vi "calc max motor speed.vi"(10 "DRIVE\nwheel diam (in)":dbl, 11 "swerve motor":T1 {"gear ratio" format="%_5f"; "MOTOR SELECT" items=["REV NEO"=5676, "REV NEO 550"=11000, "VEX Falcon"=6380, "WC Kraken"=6000]}) -> (2 "mav vel (fps)":dbl, 3 "max rpm":dbl)   [LabVIEW 2023]
uses:
  ctrl defs/ctrl swerve motor.ctl
  ctrl defs/ctrl MOTOR SELECT.ctl
  <vilib>/Rock Robotics/WPI/ThirdParty/REV Robotics/REVLib/Typedef/Spark MAX Idle Mode.ctl
  ctrl defs/ctrl Spark MAX current limiting.ctl
  ctrl defs/ctrl motor PIDF coefficients.ctl
  <vilib>/Rock Robotics/WPI/ThirdParty/REV Robotics/REVLib/Typedef/Spark MAX Smart Motion Parameters.ctl
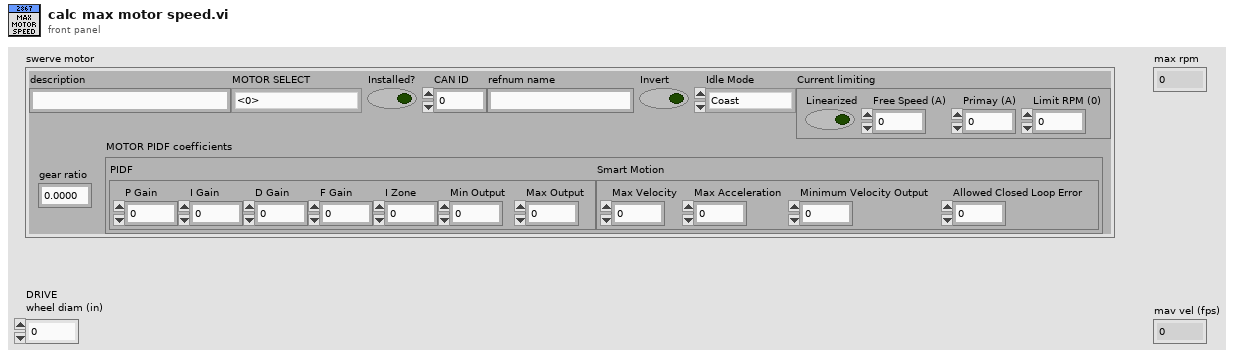
[diagram p1: front panel]
types:
  T1 = typedef "ctrl swerve motor.ctl" = cluster{"description":string, "MOTOR SELECT":T2, "Installed?":bool, "CAN ID":u8, "refnum name":string, "Invert":bool, "Idle Mode":T3, "Current limiting":T4, "MOTOR PIDF coefficients":T5, "gear ratio":dbl}
  T2 = typedef "ctrl MOTOR SELECT.ctl" = i16
  T3 = typedef "Spark MAX Idle Mode.ctl" = enum16{"Coast", "Brake"}
  T4 = typedef "ctrl Spark MAX current limiting.ctl" = cluster{"Linearized":bool, "Free Speed (A)":dbl, "Primay (A)":dbl, "Limit RPM (0)":u32}
  T5 = typedef "ctrl motor PIDF coefficients.ctl" = cluster{"PIDF":cluster{"P Gain":dbl, "I Gain":dbl, "D Gain":dbl, "F Gain":dbl, "I Zone":dbl, "Min Output":dbl, "Max Output":dbl}, "Smart Motion":T6}
  T6 = typedef "Spark MAX Smart Motion Parameters.ctl" = cluster{"Max Velocity":dbl, "Max Acceleration":dbl, "Minimum Velocity Output":dbl, "Allowed Closed Loop Error":dbl}
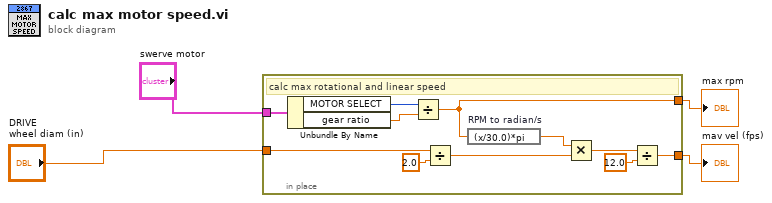
[diagram p0: block diagram]
diagram:
  n1 = in-place {
    in-place-border: "swerve motor" -> [w15]
    in-place-border: [w12] -> w3
    in-place-border: "DRIVE\nwheel diam (in)" -> [w11]
    in-place-border: [w6] -> w4
    # "calc max rotational and linear speed"
    n2 = Unbundle By Name(w15) -> ("MOTOR SELECT"=w14:T2, "gear ratio"=w13:dbl)
    n3 = Divide(x=w14, y=w13) -> (x/y=w12:dbl)
    n4 = Divide(x=w11, y=2.0) -> (x/y=w8:dbl)
    n5 = expression code="(x/30.0)*pi" "RPM to radian/s"(w12) -> (w9:dbl)
    n6 = Multiply(x=w9, y=w8) -> (x*y=w7:dbl)
    n7 = Divide(x=w7, y=12.0) -> (x/y=w6:dbl)
  }
  "mav vel (fps)" <- w4
  "max rpm" <- w3
